vi "LVClasse_Intensity Get Data.vi"(0 "Intensity in":refnum<class "Intensity.lvclass">, 7 "Pupil":refnum<class "Pupil.lvclass">, 11 "error in (no error)":errorcluster) -> (4 "Intensity out":refnum<class "Intensity.lvclass">, 6 "data":sgl[][](array[numeric]), 8 "Pupil (dup)":refnum<class "Pupil.lvclass">, 15 "error out":errorcluster)   [LabVIEW 2020, in "Intensity.lvclass"]
doc: "Phase values buffer and pupil getter.\n\n--------------------------------------------------------------------------------\n\n<B>PhaseIn </B> : Phase object.\n<B>PhaseOut </B> : Phase object.\n<B>buffer </B> : Phase values buffer.\n<B>Pupil </B> : pupil object.\n<B>ErrorIn </B> : Error\n<B>ErrorOut </B> : Error\n\n--------------------------------------------------------------------------------"
uses:
  Intensity.lvclass
  Pupil.lvclass
  Intensity.lvclass/Intensity.ctl
  LVClass_Pupil Read Pupil.vi
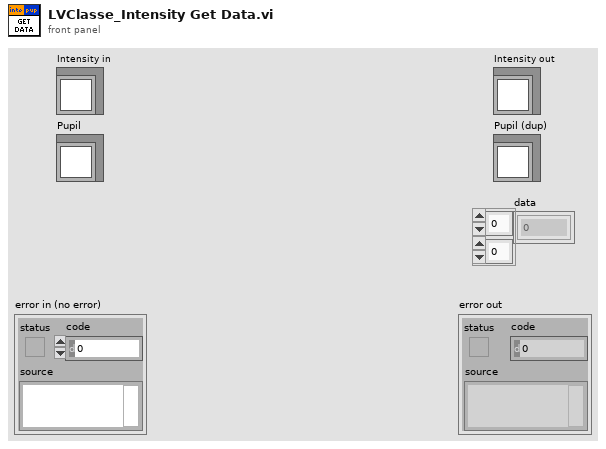
[diagram p1: front panel]
types:
  T1 = typedef "General dimensions definition.ctl" = cluster{"Size":T2, "Step":T3}
  T2 = typedef "Point2D.ctl" = cluster{"X":u32, "Y":u32}
  T3 = typedef "Point2Df.ctl" = cluster{"X":sgl, "Y":sgl}
  T4 = typedef "ClassID.ctl" = i64
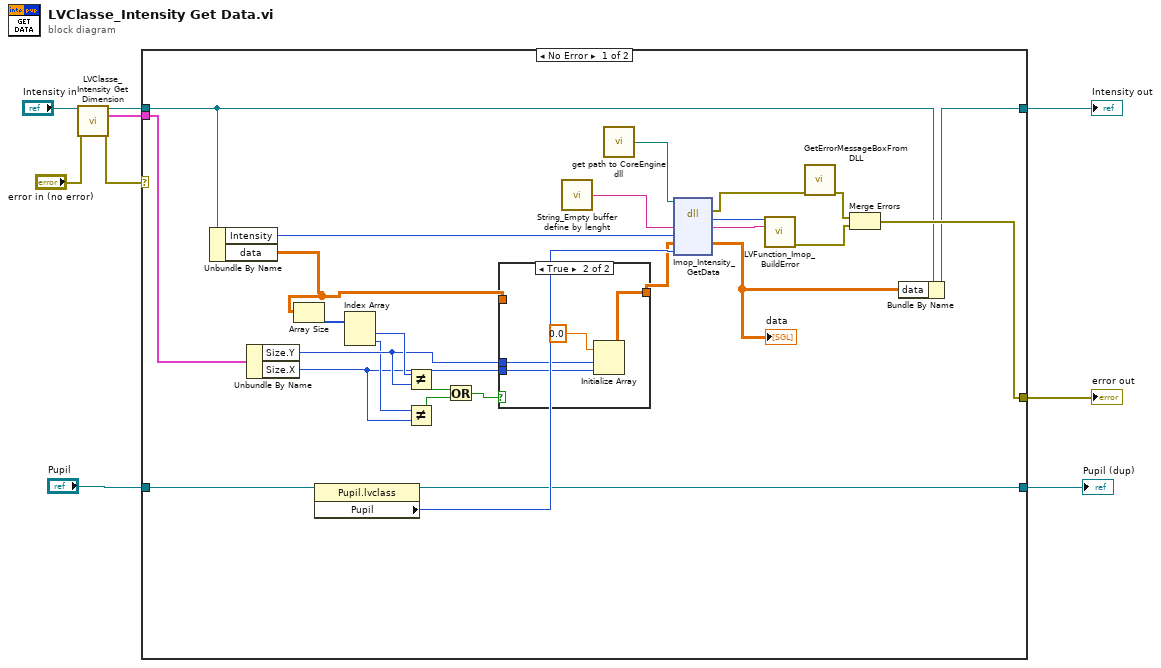
[diagram p0: block diagram]
diagram:
  n1 = call "LVClasse_Intensity Get Dimension.vi"("Intensity in"="Intensity in", "error in (no error)"="error in (no error)") -> ("Intensity out"=w6:refnum<class "Intensity.lvclass">, "Dimensions_um"=w3:T1, "error out"=w4:errorcluster)  [unwired: 11 in]
  n2 = case shown="No Error" w4 {
    selector: w4 -> [_ w43]
    tunnel: [w24 w43] -> w9
    tunnel: [w11 w42] -> w8
    tunnel: w6 -> [w12 w42]
    tunnel: w3 -> [w14 _]
    tunnel: "Pupil" -> [w29 w41]
    tunnel: [w27 w41] -> w1
    frame No Error {
      n3 = Unbundle By Name(w12) -> ("Intensity"=w30:T4, "data"=w15:sgl[][])
      n4 = Unbundle By Name(w14) -> ("Size.Y"=w21:u32, "Size.X"=w19:u32)
      n5 = Array Size(array=w15) -> (size(s)=w23:i32[])
      n6 = property class="Pupil.lvclass"(reference=w29) -> (reference out=w27:refnum<class "Pupil.lvclass">, "Pupil"=w28:T4)  [unwired: 1 in, 1 out]
      n7 = Index Array(array=w23) -> (element #1=w22:i32, element #2=w20:i32)  [unwired: 2 in]
      n8 = Not Equal?(x=w22, y=w21) -> (x != y?=w18:bool)
      n9 = Not Equal?(x=w20, y=w19) -> (x != y?=w17:bool)
      n10 = Or(x=w18, y=w17) -> (x .or. y?=w16:bool)
      n11 = case shown="True" w16 {
        tunnel: [w36 w38] -> w13
        tunnel: w21 -> [_ w40]
        tunnel: w19 -> [_ w39]
        tunnel: w15 -> [w36 _]
        frame False {
        }
        frame True {
          n12 = Initialize Array(sgl 0.0, w40, w39) -> (w38:sgl[][])
        }
      }
      n13 = call "String_Empty buffer define by lenght.vi"() -> ("Empty buffer"=w33:string)  [unwired: 1 in]
      n14 = call "get path to CoreEngine dll.vi"() -> ("path to wavekit library"=w32:path)  [unwired: 14 in, 1 out]
      n15 = dll-call lib="D:/2_trunk/Soft_haso/ImOpCoreEngine4_LV2011/DLLs/ImopEngine4_vc100.dll" fn="Imop_Intensity_GetData"(path in=w32, "message"=w33, "intensity"=w30, "data"=w13, "pupil"=w28) -> (error out=w31:errorcluster, "return type"=w35:i32, "message"=w34:string, "data"=w10:sgl[][])  [unwired: 4 in, 1 out]
      "data" <- w10
      n16 = call "LVFunction_Imop_BuildError.vi"("code"=w35, "String to Prepend to source (\"\")"=w34) -> ("error out"=w25:errorcluster)  [unwired: 13 in]
      n17 = call "GetErrorMessageBoxFromDLL.vi"("error IN"=w31) -> ("error OUT"=w26:errorcluster)  [unwired: 10 in]
      n18 = Merge Errors(w26, w25) -> (w24:errorcluster)
      n19 = Bundle By Name(cluster=w12, "data"=w10) -> (w11:refnum<class "Intensity.lvclass">)
    }
    frame Error {
    }
  }
  "error out" <- w9
  "Intensity out" <- w8
  "Pupil (dup)" <- w1
